vi "Test_SQLQueryVIM2DI64_WorksNoError.vi"(8 "error in (no error)":errorcluster, 11 "TestCase in":refnum<class "Test mysql.lvclass">) -> (0 "error out":errorcluster, 3 "TestCase out":refnum<class "Test mysql.lvclass">)   [LabVIEW 2020, in "DataBase_mysql_Tests.lvlib" / "Test mysql.lvclass"]
uses:
  Test mysql.lvclass
  98ffd0c8-4361-48ce-8721-6d705661544a.vi
  98ffd0c8-4361-48ce-8721-6d705661544a.vi/34fb6e58-d5df-4b5d-8e4a-f2f1e82f356e.vi
  98ffd0c8-4361-48ce-8721-6d705661544a.vi/059538b5-1ca7-4933-9232-b8f62955952d.vi
  <vilib>/Utility/error.llb/Error Cluster From Error Code.vi
  externals/mysql/Source/mysql.net/mysql.lvclass
  <vilib>/addons/_JKI Toolkits/VI Tester/TestCase.llb/TestCase.lvclass
  C:/Program Files/National Instruments/LabVIEW 2020/vi.lib/addons/_JKI Toolkits/VI Tester/TestCase.llb/TestCase.lvclass
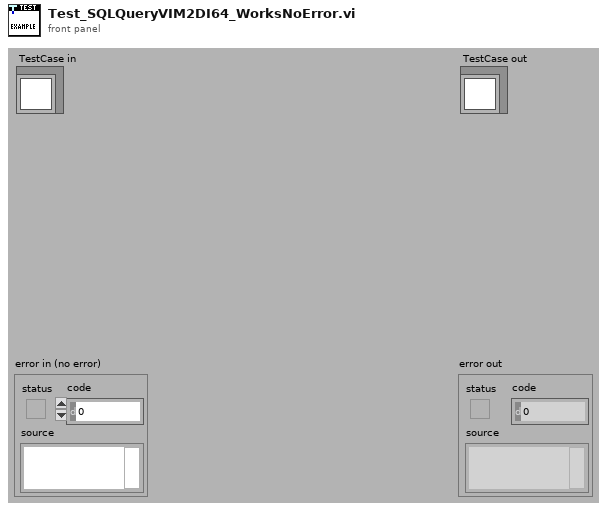
[diagram p1: front panel]
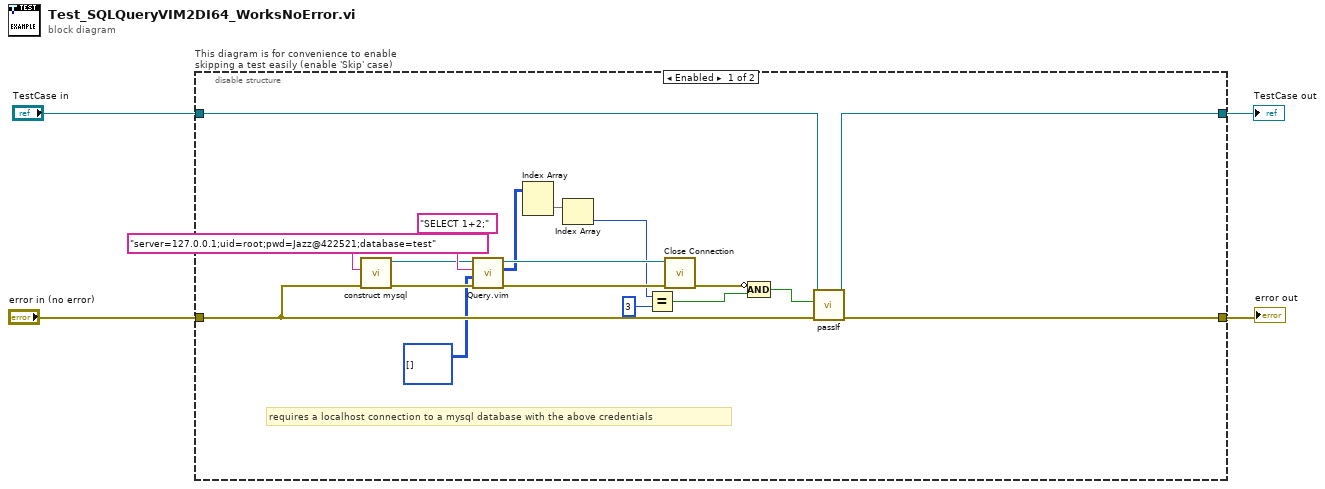
[diagram p0: block diagram]
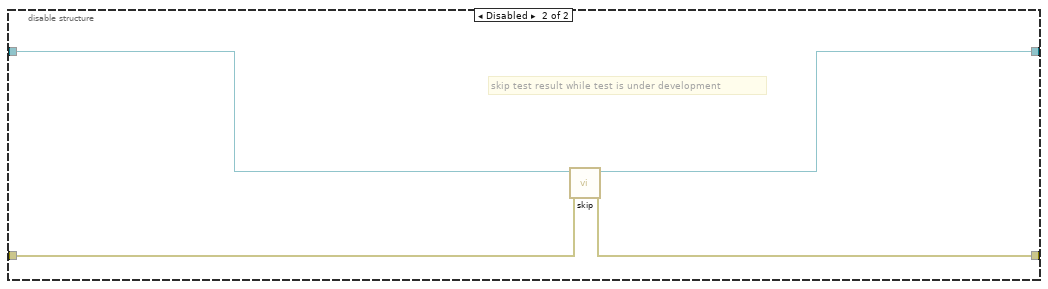
[diagram p2: hidden frame]
diagram:
  n1 = disable-structure "This diagram is for convenience to enable skipping a test easily (enable 'Skip' case)" shown="Enabled" {
    disable-tunnel: "TestCase in" -> [w22 w26]
    disable-tunnel: [w21 w24] -> w1
    disable-tunnel: [w20 w25] -> w3
    disable-tunnel: "error in (no error)" -> [w18 w23]
    frame Enabled {
      # "requires a localhost connection to a mysql database with the above credentials"
      n2 = call "construct mysql.vi"("error in (no error)"=w18, "Connection string"="server=127.0.0.1;uid=root;pwd=Jazz@422521;database=test") -> ("error out"=w12:errorcluster, "mysql out"=w5:refnum<class "mysql.lvclass">)  [unwired: 8 in]
      n3 = call "Query.vim"("error in (no error)"=w12, "Type and Default"=i64[][] [], "Query string"="SELECT 1+2;", "IDatabase in"=w5) -> ("error out"=w11:errorcluster, "Result"=w9:i64[][], "IDatabase out"=w13:refnum<class "mysql.lvclass">)  [unwired: 5 in]
      n4 = Index Array(array=w9) -> (element=w7:i64[])  [unwired: 2 in]
      n5 = Index Array(array=w7) -> (element=w6:i64)  [unwired: 1 in]
      n6 = Equal?(x=w6, y=i64 3) -> (x = y?=w14:bool)
      n7 = call-dynamic "Close Connection.vi"("error in (no error)"=w11, "mysql in"=w13) -> ("error out"=w17:errorcluster)  [unwired: 8 in, 1 out]
      n8 = Compound Arithmetic op=AND(invert w17, w14) -> (w16:bool)
      n9 = call-dynamic "passIf.vi"("error in (no error)"=w18, "pass"=w16, "TestCase in"=w22) -> ("error out"=w20:errorcluster, "TestCase out"=w21:refnum<class "Test mysql.lvclass">)  [unwired: 7 in]
    }
    frame Disabled {
      # "skip test result while test is under development"
      n10 = call <vilib>:"skip.vi"("error in (no error)"=w23, "TestCase in"=w26) -> ("error out"=w25:errorcluster, "TestCase out"=w24:refnum<class "Test mysql.lvclass">)  [unwired: 8 in]
    }
  }
  "error out" <- w3
  "TestCase out" <- w1
